vi "Request Supported.vi"(8 "error in (no error)":errorcluster, 10 "Request":refnum<class "Request.lvclass">, 11 "FormAuthentication in":refnum<class "FormAuthentication.lvclass">) -> (0 "error out":errorcluster, 2 "Supported":bool, 3 "FormAuthentication out":refnum<class "FormAuthentication.lvclass">)   [LabVIEW 2020, in "HTTP Server.lvlib" / "FormAuthentication.lvclass"]
uses:
  FormAuthentication.lvclass
  lv-http-util/HTTP Utils/Request/Request.lvclass
  FormAuthentication.lvclass/FormAuthentication.ctl
  lv-uri/URI/URI/URI.lvclass
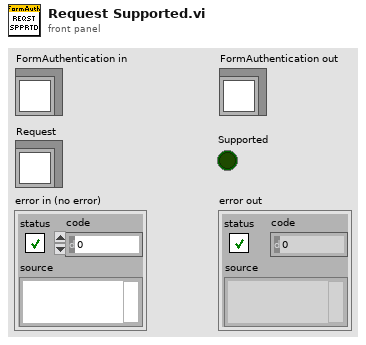
[diagram p1: front panel]
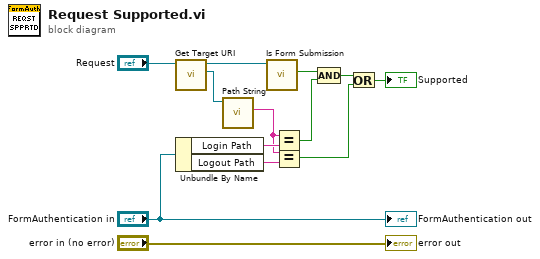
[diagram p0: block diagram]
diagram:
  n1 = call "Get Target URI.vi"("Request in"="Request") -> ("Target URI"=w10:refnum<class "URI.lvclass">, "Request out"=w11:refnum<class "Request.lvclass">)  [unwired: 8 in, 1 out]
  n2 = Unbundle By Name("FormAuthentication in") -> ("Login Path"=w8:string, "Logout Path"=w4:string)
  n3 = call "Path String.vi"("URI in"=w10) -> ("Path String"=w3:string)  [unwired: 9 in, 1 out]
  n4 = call "Is Form Submission.vi"("Request in"=w11) -> ("Is Form Submission?"=w7:bool)  [unwired: 8 in, 2 out]
  n5 = Equal?(x=w3, y=w8) -> (x = y?=w6:bool)
  n6 = Equal?(x=w3, y=w4) -> (x = y?=w1:bool)
  n7 = Compound Arithmetic op=AND(w7, w6) -> (w5:bool)
  n8 = Or(x=w5, y=w1) -> (x .or. y?=→"Supported":bool)
  "error out" <- "error in (no error)"
  "FormAuthentication out" <- "FormAuthentication in"
